vi "String2BCCD.vi"(11 "String":string) -> (3 "BCD Int":i64)   [LabVIEW 2020]
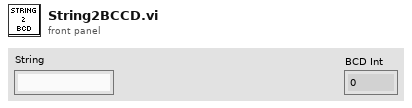
[diagram p1: front panel]
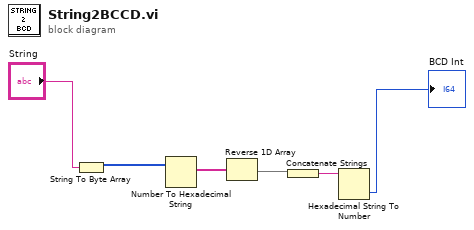
[diagram p0: block diagram]
diagram:
  n1 = String To Byte Array(string="String") -> (unsigned byte array=w6:u8[])
  n2 = Number To Hexadecimal String(2:w6) -> (0:w4:string[])  [unwired: 1 in]
  n3 = Reverse 1D Array(array=w4) -> (reversed array=w3:string[])
  n4 = Concatenate Strings(w3) -> (w5:string)
  n5 = Hexadecimal String To Number(string=w5) -> (number=→"BCD Int":u32)  [unwired: 2 in, 1 out]
